vi "UE9 Quadrature with Z-phase.vi"(8 "error in":errorcluster) -> (0 "error out":errorcluster)   [LabVIEW 2021]
panel:
  in  "DeviceType":u16(ring)=1 items=["LJ_dtU3", "LJ_dtUE9"]
  in  "Stop":bool
  in  "Reset Count":bool
  out "Quadrature Count":i32
  in  "FirstFound":bool=TRUE
  in  "Address":string="1"
  in  "ConnectionType":u16(ring) items=["LJ_ctUSB", "LJ_ctETHERNET"]
  out "Error Message":string
  # "Demonstrates 1 quadrature input, which uses two timer channels for phases A and B (FIO0 and FIO1 in this case).\nIf you don't have a quadrature signal source handy, you can connect wires to GND, and tap these wires on FIO0\nand FIO1 to simulate quadrature.\n\nWith Control firmware V2.06, support for Z-phase reset was added.  If enabled for a particular timer, the Z-phase\nstate is read during the interrupt for a rising edge on that timer.  If high, the quadrature count is reset.  The\nTimer Value passed in during configuration is used to enable and configure Z-phase reset:\n\nBit 7:  Enable Z-phase reset.\nBits 0-6:  Digital I/O used to read Z-phase.\n\nThis example passes a value of d130 (b10000010) for Timer0, so the Z-phase should be connected to FIO2 and\nis checked just after a rising edge on the A-phase."
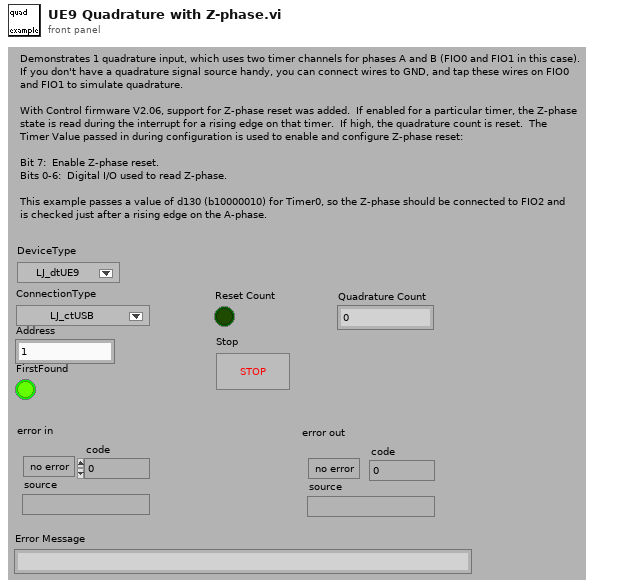
[diagram p1: front panel]
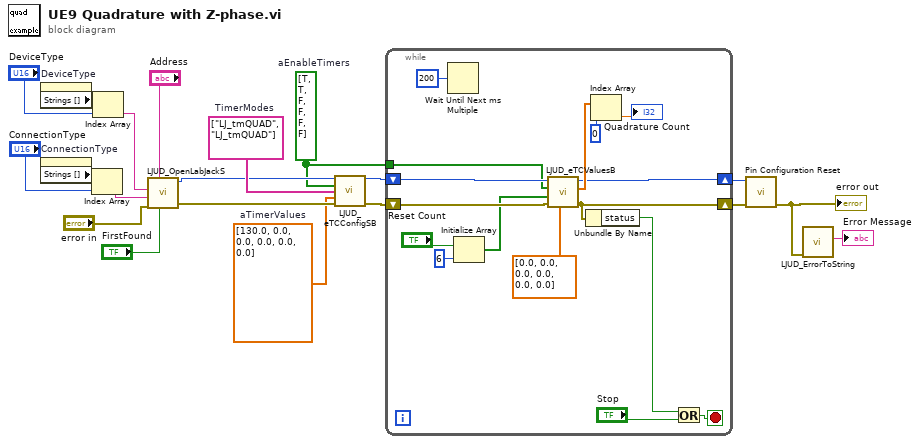
[diagram p0: block diagram]
diagram:
  w1 = dbl[] [130.0, 0.0, 0.0, 0.0, 0.0, 0.0]  # aTimerValues
  w2 = bool[] [TRUE, TRUE, FALSE, FALSE, FALSE, FALSE]  # aEnableTimers
  w8 = string[] ["LJ_tmQUAD", "LJ_tmQUAD"]  # TimerModes
  n1 = property on="DeviceType" class="Ring (strict)"() -> ("Strings []"=w11:string[])  [unwired: 2 in, 2 out]
  n2 = property on="ConnectionType" class="Ring (strict)"() -> ("Strings []"=w13:string[])  [unwired: 2 in, 2 out]
  n3 = Index Array(array=w13, index="ConnectionType") -> (element=w12:string)
  n4 = Index Array(array=w11, index="DeviceType") -> (element=w9:string)
  n5 = call "LJUD_OpenLabJackS.vi"("FirstFound"="FirstFound", "Address"="Address", "error in"="error in", "ConnectionType"=w12, "DeviceType"=w9) -> ("error out"=w6:errorcluster, "Handle"=w7:i32)  [unwired: 4 in, 1 out]
  n6 = call "LJUD_eTCConfigSB.vi"("Handle In"=w7, "aEnableTimers"=w2, "aTimerModes"=w8, "aTimerValues"=w1, "error in"=w6) -> ("Handle Out"=w15:i32, "error out"=w16:errorcluster)  [unwired: 9 in]
  n7 = while {
    tunnel: w2 -> [w21]
    shift-left: w16 -> [w32]
    shift-right: [w30] -> w4
    shift-left: w15 -> [w33]
    shift-right: [w31] -> w5
    stop <- w29 stop-if-true
    n8 = Wait Until Next ms Multiple(millisecond multiple=u32 200) -> ()  [unwired: 1 out]
    n9 = Initialize Array("Reset Count", 6 ("Dimension Size")) -> (w23:bool[])
    n10 = call "LJUD_eTCValuesB.vi"("aTimerValues Write"=dbl[] [0.0, 0.0, 0.0, 0.0, 0.0, 0.0] ("TimerValues"), "error in"=w32, "aUpdateResetTimers"=w23, "aReadTimers"=w21, "Handle In"=w33) -> ("error out"=w30:errorcluster, "aTimerValues Read"=w34:dbl[], "Handle Out"=w31:i32)  [unwired: 3 in, 1 out]
    n11 = Unbundle By Name(w30) -> ("status"=w28:bool)
    n12 = Index Array(array=w34, index=0 ("Index")) -> (element=→"Quadrature Count":dbl)
    n13 = Or(x=w28, y="Stop") -> (x .or. y?=w29:bool)
  }
  n14 = call "Pin Configuration Reset.vi"("error in"=w4, "Handle In"=w5) -> ("error out"=w3:errorcluster)  [unwired: 8 in, 1 out]
  "error out" <- w3
  n15 = call "LJUD_ErrorToString.vi"("error in"=w3) -> ("String"=→"Error Message":string)  [unwired: 10 in]
